vi "Set Pipe Mode.vi"(8 "error in":errorcluster, 10 "Variable Pipe Mode? (F)":bool, 11 "GOLPI ref. in":T1={"pipe handle"={"lv_proc.dll file path"=path "", "process instance handle"=[], "debug mode"=FALSE, "debug data"=[]}, "fast read timeout [ms]"=500, "fast read settle time [ms]"=10, "fast read to multiple [ms]"=1, "max elements per input line"=100, "slow read timeout [ms]"=5000, "stdin double format specifier"="", "max elements per stdout output column"=100, "console mode bitstream"=FALSE, "bitstream first read timeout [ms]"=1000, "bitstream read timeout [ms]"=50, "struct transfer possible"=FALSE, "matlab mode"=FALSE, "var pipe write timeout [ms]"=5000, "variable pipe mode"=FALSE, "variable pipe buffer size [Bytes]"=10000000, "variable pipe block size [Bytes]"=1000000} {"variable pipe block size [Bytes]" format="%.0p"; "variable pipe buffer size [Bytes]" format="%.0p"}) -> (0 "error out":errorcluster, 3 "GOLPI ref. out":T1={"pipe handle"={"lv_proc.dll file path"=path "", "process instance handle"=[], "debug mode"=FALSE, "debug data"=[]}, "fast read timeout [ms]"=500, "fast read settle time [ms]"=10, "fast read to multiple [ms]"=1, "max elements per input line"=100, "slow read timeout [ms]"=5000, "stdin double format specifier"="", "max elements per stdout output column"=100, "console mode bitstream"=FALSE, "bitstream first read timeout [ms]"=1000, "bitstream read timeout [ms]"=50, "struct transfer possible"=FALSE, "matlab mode"=FALSE, "var pipe write timeout [ms]"=5000, "variable pipe mode"=FALSE, "variable pipe buffer size [Bytes]"=10000000, "variable pipe block size [Bytes]"=1000000} {"variable pipe block size [Bytes]" format="%.0p"; "variable pipe buffer size [Bytes]" format="%.0p"})   [LabVIEW 2020, in "GOLPI library.lvlib"]
doc: "Set variable pipe transfer mode (only for GNU Octave, for Matlab not supported/needed). When set, data are transfered from Octave to LabVIEW using golpi GNU Octave package. This package pipe functions transfer variables via windows named pipes which is faster than via console. First this VI tries to install GNU Octave package golpi and compile C++ functions handling the pipe transfers. Than package is loaded and VI checks if functions are available in current GNU Octave instance. If not error error is generated. Note the compilation of C++ code is unpredictable with GNU Octave, so it may not succed depending on particular version and installation. \n\n---\nGOLPI works only with lv_proc.dll library, which is part of vipm package or should be delivered together with packed library. Placement of this dll is selected in terminal of Start GNU Octave.vi."
uses:
  GOLPI library.lvlib
  GOLPI reference Type Def.ctl
  LV Process source distribution/Pipe Handle.ctl
  Private/Type Definitions/Custom Error Codes Enum Type Def.vi
  <vilib>/regexp/Match Regular Expression.xnode
  LV Process source distribution/LV Process library.lvlib
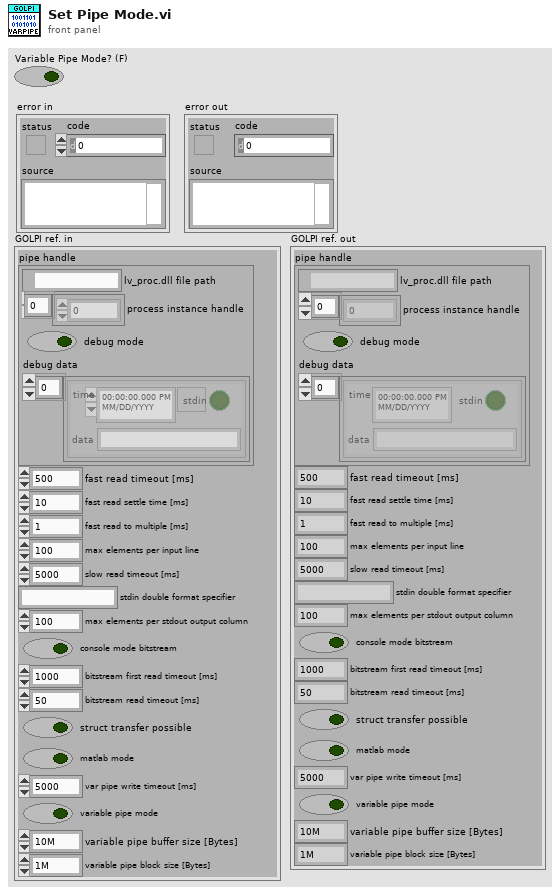
[diagram p1: front panel]
types:
  T1 = typedef "GOLPI library.lvlib/GOLPI reference Type Def.ctl" = cluster{"pipe handle":T2, "fast read timeout [ms]":u32, "fast read settle time [ms]":u32, "fast read to multiple [ms]":u32, "max elements per input line":u32, "slow read timeout [ms]":u32, "stdin double format specifier":string, "max elements per stdout output column":u32, "console mode bitstream":bool, "bitstream first read timeout [ms]":u32, "bitstream read timeout [ms]":u32, "struct transfer possible":bool, "matlab mode":bool, "var pipe write timeout [ms]":u32, "variable pipe mode":bool, "variable pipe buffer size [Bytes]":u32, "variable pipe block size [Bytes]":u32}
  T2 = typedef "LV Process library.lvlib/Pipe Handle.ctl" = cluster{"lv_proc.dll file path":path, "process instance handle":u32[], "debug mode":bool, "debug data":cluster{"time":timestamp, "stdin":bool, "data":string}[]}
  T3 = typedef "GOLPI library.lvlib/Custom Error Codes Enum Type Def.vi" = enum16{"no error", "00 working directory PAR1 missing", "01 octave binary PAR1 missing", "02 octave report error PAR1", "03 empty output last cmd PAR1", "04 missing temporary file PAR1", "05 pwd PAR 1 not exist", "06 oct package not installed", "07 octave default binary missing", "10 var PAR1 not string, vect", "11 var PAR1 not num, scal, ~compl", "12 var PAR1 not num, scal, compl", "13 var PAR1 not num, vect, ~compl", "14 var PAR1 not num, vect, compl", "15 var PAR1 not num, mat, ~compl", "16 var PAR1 not num, mat, ~compl", "30 read timeout", "60 bitstream transport failed", "61 bitstream decode error PAR1", "62 bitstream cannot be set", "70 struct transfer not possible", "80 struct: cluster elem. PAR1 not implem.", "81 struct: structure field PAR1 not implem.", "82 struct: size mismatch of PAR1", "83 struct: type mismatch of PAR1", "98 internal error", "99 not finished", "90 Not supported in Matlab mode", "91 Matlab variable transfer error", "92 Matlab Script Error", "100 Variable Pipe Mode cannot be set"}
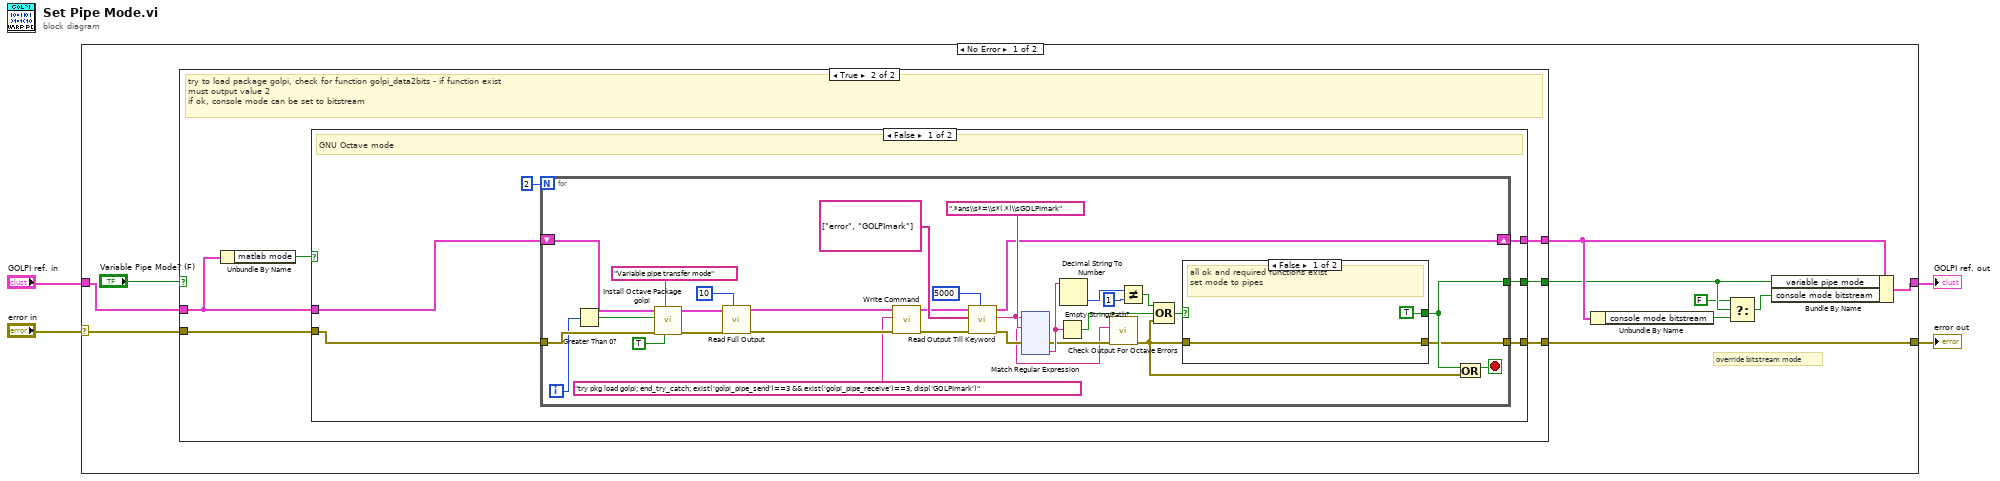
[diagram p0: block diagram]
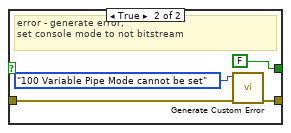
[diagram p3: hidden frame]
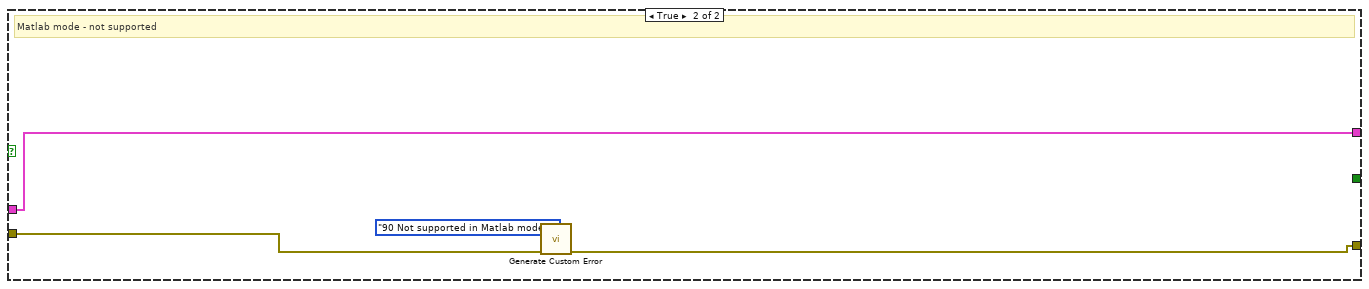
[diagram p4: hidden frame]
diagram:
  n1 = case shown="No Error" "error in" {
    selector: "error in" -> [w11 w188]
    tunnel: "GOLPI ref. in" -> [w12 w187]
    tunnel: [w14 w187] -> w3
    tunnel: [w10 w188] -> w1
    frame No Error {
      # "override bitstream mode"
      n2 = case shown="True" "Variable Pipe Mode? (F)" {
        selector: "Variable Pipe Mode? (F)" -> [w17 _]
        tunnel: [w17 w22] -> w8
        tunnel: w12 -> [w16 w19]
        tunnel: w11 -> [w15 w20]
        tunnel: [w15 w21] -> w10
        tunnel: [w16 w23] -> w9
        frame False {
          # "set console mode - this can be done withnout any checks or conditions"
        }
        frame True {
          # "try to load package golpi, check for function golpi_data2bits - if function exist\nmust output value 2\nif ok, console mode can be set to bitstream"
          n3 = Unbundle By Name(w19) -> ("matlab mode"=w18:bool)
          n4 = case shown="False" w18 {
            tunnel: [w29 w184] -> w23
            tunnel: [w28 _] -> w22
            tunnel: [w27 w183] -> w21
            tunnel: w20 -> [w26 w186]
            tunnel: w19 -> [w25 w184]
            frame False {
              # "GNU Octave mode"
              n5 = for {
                N: 2 -> [_]
                tunnel: [w35] -> w28
                shift-right: [w47] -> w29
                shift-left: w25 -> [w38]
                tunnel: w26 -> [w41]
                tunnel: [w33] -> w27
                i -> [w32]
                stop <- w34 stop-if-true
                n6 = Greater Than 0?(x=w32) -> (x > 0?=w31:bool)
                n7 = call "Install Octave Package golpi.vi"("Verbose? (T)"=TRUE, "Feature name"="Variable pipe transfer mode", "error in"=w41, "force reinstall? (F)"=w31, "GOLPI ref. in"=w38) -> ("error out"=w40:errorcluster, "GOLPI ref. out"=w39:T1)  [unwired: 5 in]
                n8 = call "Read Full Output.vi"("timeout [ms]"=u32 10, "error in"=w40, "GOLPI ref. in"=w39) -> ("error out"=w59:errorcluster, "GOLPI ref. out"=w60:T1)  [unwired: 5 in, 2 out]
                n9 = call "Write Command.vi"("error in"=w59, "command"="try pkg load golpi; end_try_catch; exist('golpi_pipe_send')==3 && exist('golpi_pipe_receive')==3, disp('GOLPImark')", "GOLPI ref. in"=w60) -> ("error out"=w50:errorcluster, "GOLPI ref. out"=w48:T1)  [unwired: 7 in]
                n10 = call "Read Output Till Keyword.vi"("timeout [ms]"=u32 5000, "error in"=w50, "keywords"=string[] ["error", "GOLPImark"], "GOLPI ref. in"=w48) -> ("error out"=w49:errorcluster, "read buffer"=w42:string, "GOLPI ref. out"=w47:T1)  [unwired: 4 in, 1 out]
                n11 = xnode "Match Regular Expression"("input string"=w42, "regular expression"=".*ans\\s*=\\s*(.*)\\sGOLPImark", "error in"=w49) -> ("error out"=w51:errorcluster, "submatch 1"=w54:string)  [unwired: 3 in, 4 out]
                n12 = Empty String/Path?(string/path=w54) -> (empty?=w55:bool)
                n13 = Decimal String To Number(string=w54) -> (number=w43:i32)  [unwired: 2 in, 1 out]
                n14 = call "Check Output For Octave Errors.vi"("error in"=w51, "read buffer"=w42) -> ("error out"=w30:errorcluster)  [unwired: 9 in]
                n15 = Not Equal?(x=w43, y=1) -> (x != y?=w52:bool)
                n16 = Compound Arithmetic op=OR(w52, w55, w30) -> (w45:bool)
                n17 = case shown="False" w45 {
                  tunnel: [TRUE FALSE] -> w35
                  tunnel: [w62 w64] -> w33
                  tunnel: w30 -> [w62 w65]
                  frame False {
                    # "all ok and required functions exist\nset mode to pipes"
                  }
                  frame True {
                    # "error - generate error, \nset console mode to not bitstream"
                    n18 = call "Generate Custom Error.vi"("error in"=w65, "GOLPI error"=Custom_Error_Codes_Enum_Type_Def.vi."100 Variable Pipe Mode cannot be set") -> ("error out"=w64:errorcluster)  [unwired: 9 in]
                  }
                }
                n19 = Compound Arithmetic op=OR(w35, w30) -> (w34:bool)
              }
            }
            frame True {
              # "Matlab mode - not supported"
              n20 = call "Generate Custom Error.vi"("error in"=w186, "GOLPI error"=Custom_Error_Codes_Enum_Type_Def.vi."90 Not supported in Matlab mode") -> ("error out"=w183:errorcluster)  [unwired: 9 in]
            }
          }
        }
      }
      n21 = Unbundle By Name(w9) -> ("console mode bitstream"=w7:bool)
      n22 = Select(t=FALSE, s=w8, f=w7) -> (s? t:f=w6:bool)
      n23 = Bundle By Name(cluster=w9, "variable pipe mode"=w8, "console mode bitstream"=w6) -> (w14:T1)
    }
    frame Error {
    }
  }
  "error out" <- w1
  "GOLPI ref. out" <- w3
